vi "sub_Text_To_Bitstream.vi"(9 "Packet\nMessage Length (bits)":i32, 11 "text":string) -> (1 "File Length (bits)":i32, 3 "message bitstream":i8[](array[numeric]), 4 "Number of Packets":i32)   [LabVIEW 2013]
panel:
  out "Array":i8[][](array[numeric])
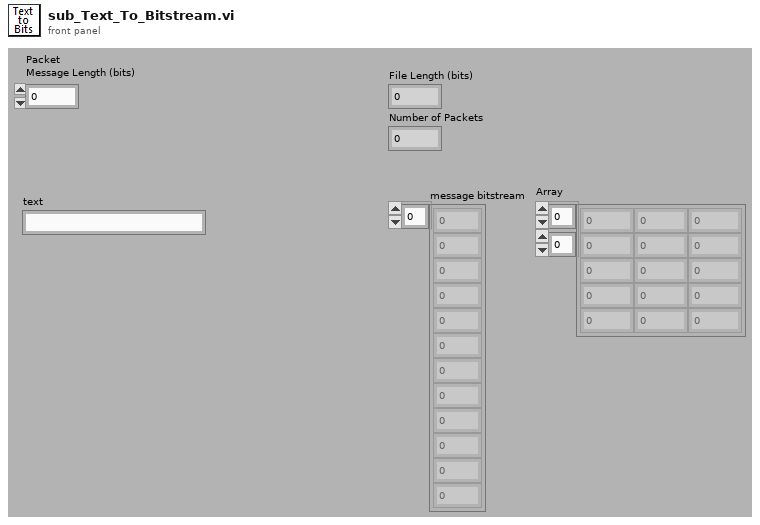
[diagram p1: front panel]
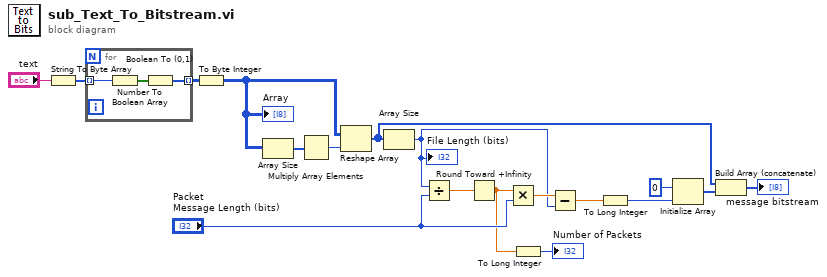
[diagram p0: block diagram]
diagram:
  n1 = String To Byte Array(string="text") -> (unsigned byte array=w17:u8[])
  n2 = for {
    tunnel: w17 -> [w21] mode=indexing
    tunnel: [w19] -> w16 mode=indexing
    n3 = Number To Boolean Array(number=w21) -> (Boolean array=w20:bool[])
    n4 = Boolean To (0,1)(Boolean=w20) -> (0, 1=w19:i16[])
  }
  n5 = To Byte Integer(number=w16) -> (8bit integer=w1:i8[][])
  "Array" <- w1
  n6 = Array Size(array=w1) -> (size(s)=w15:i32[])
  n7 = Multiply Array Elements(1:w15) -> (0:w14:i32)
  n8 = Reshape Array(w1, w14) -> (w4:i8[])
  n9 = Array Size(array=w4) -> (size(s)=w10:i32)
  "File Length (bits)" <- w10
  n10 = Divide(x=w10, y="Packet\nMessage Length (bits)") -> (x/y=w12:dbl)
  n11 = Round Toward +Infinity(x=w12) -> (ceil(x): smallest int >= x=w7:dbl)
  n12 = Multiply(x=w7, y="Packet\nMessage Length (bits)") -> (x*y=w11:dbl)
  n13 = To Long Integer(number=w7) -> (32bit integer=→"Number of Packets":i32)
  n14 = Subtract(x=w11, y=w10) -> (x-y=w9:dbl)
  n15 = To Long Integer(number=w9) -> (32bit integer=w5:i32)
  n16 = Initialize Array(i8 0 ("element"), w5) -> (w3:i8[])
  n17 = Build Array (concatenate)(w4, w3) -> (→"message bitstream":i8[])
